vi "On Download Starting.vi"(8 "error in (no error)":errorcluster, 10 "DownloadOperation":refnum<k24>, 11 "WebView2 Event Filter Interface in":refnum<class "WebView2 Event Filter Interface.lvclass">) -> (0 "error out":errorcluster, 2 "Response":T1)   [LabVIEW 2025, in "WebView2.lvlib" / "WebView2 Event Filter Interface.lvclass"]
uses:
  WebView2 Event Filter Interface.lvclass
  E:/Labview/LV 2023/PPL/PPL Builder/Libs/LV-WebView2/Source/Libs/Microsoft.Web.WebView2.Core.dll
  Libs/Microsoft.Web.WebView2.Core.dll
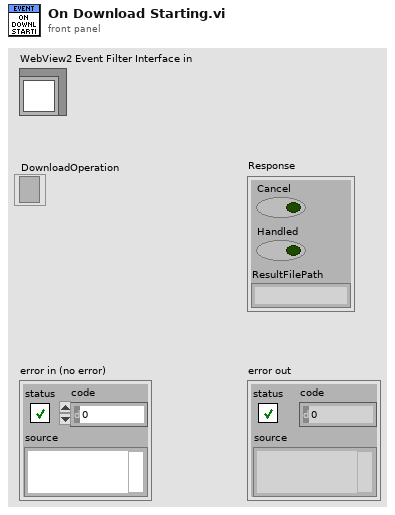
[diagram p1: front panel]
types:
  T1 = cluster{"Cancel":bool, "Handled":bool, "ResultFilePath":string}
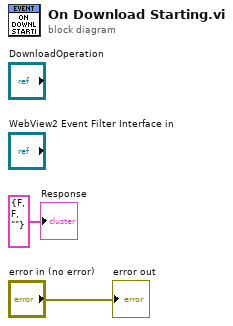
[diagram p0: block diagram]
diagram:
  "error out" <- "error in (no error)"
  "Response" <- T1 {"Cancel"=FALSE, "Handled"=FALSE, "ResultFilePath"=""} ("Response")
